vi "Test Instrument.vi"(0 "Instrument Prop In":T1={"Public"={"Column Name"=[], "Trace Color"=[]}, "Private"={"Path"=path "", "VI Refnum"=refnum, "Name"="", "# of Values"=0, "Scale Factors"=[], "Display"=[], "Offset"=[1.0]}} {"Private"."Offset" format="%^_3e"; "Private"."Scale Factors" format="%^_3e"}, 1 "Array":dbl[](array[numeric])) -> (2 "Instrument Prop Out":T1={"Public"={"Column Name"=[], "Trace Color"=[]}, "Private"={"Path"=path "", "VI Refnum"=refnum, "Name"="", "# of Values"=0, "Scale Factors"=[], "Display"=[], "Offset"=[1.0]}} {"Private"."Offset" format="%^_3e"; "Private"."Scale Factors" format="%^_3e"}, 3 "Array 2":dbl[](array[numeric]), 4 "Stop":bool)   [LabVIEW 2020]
uses:
  Sub Controls/Instrument Properties.ctl
  Sub Controls/Public.ctl
  Sub Controls/Private.ctl
  Sub Controls/Instrument Ref.ctl
  Sub Controls/SystemCheckBox-resize.ctl
  Sub Controls/Instrument Actions.ctl
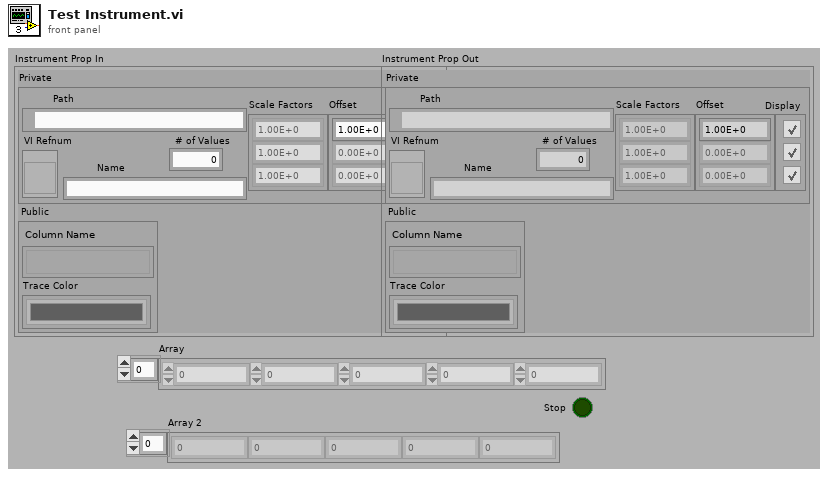
[diagram p1: front panel]
types:
  T1 = typedef "Instrument Properties.ctl" = cluster{"Public":T2, "Private":T3}
  T2 = typedef "Public.ctl" = cluster{"Column Name":string[], "Trace Color":u32[]}
  T3 = typedef "Private.ctl" = cluster{"Path":path, "VI Refnum":T4, "Name":string, "# of Values":i32, "Scale Factors":dbl[], "Display":T5[], "Offset":dbl[]}
  T4 = typedef "Instrument Ref.ctl" = refnum<vi>
  T5 = typedef "SystemCheckBox-resize.ctl" = bool
  T6 = typedef "Instrument Actions.ctl" = enum16{"Scan", "Identify", "New", "Configure", "Initialize", "Test", "Read", "Close"}
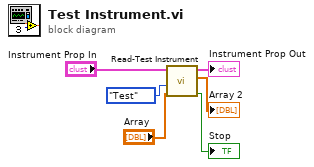
[diagram p0: block diagram]
diagram:
  n1 = call "Read-Test Instrument.vi"("Data Array In"="Array", "Action"=Instrument_Actions."Test", "Instrument Prop"="Instrument Prop In") -> ("Stop"=→"Stop":bool, "Data Array Out"=→"Array 2":dbl[], "Instrument Prop 2"=→"Instrument Prop Out":T1)  [unwired: 2 in]
